vi "QueueDriver.vi"(0 "Queue Name":string, 5 "State":T2, 7 "State[]":T2[](array[typedef]), 11 "error in (no error)":errorcluster, 13 "Operations":T1) -> (4 "Dequeued Element":T2, 15 "error out":errorcluster)   [LabVIEW 2021]
doc: "This Vi acts a queue driver performing queue operations such as enqueue and dequeue."
uses:
  Controls/State.ctl
  Controls/Operations.ctl
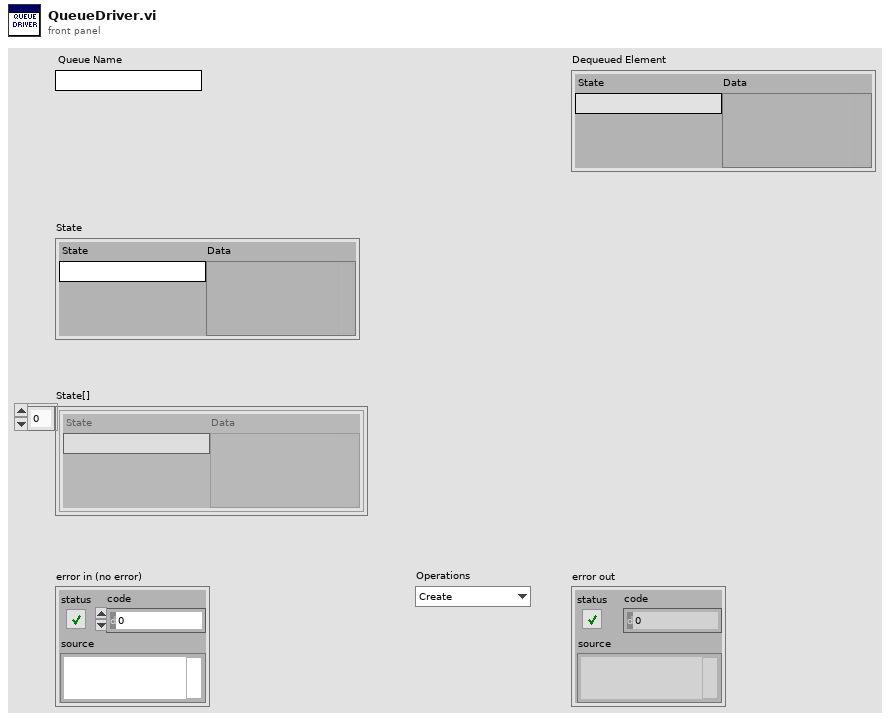
[diagram p1: front panel]
types:
  T1 = typedef "Operations.ctl" = enum16{"Create", "Enqueue", "Enqueue N", "Enstack", "Dequeue", "Flush", "Release"}
  T2 = typedef "State.ctl" = cluster{"State":string, "Data":variant}
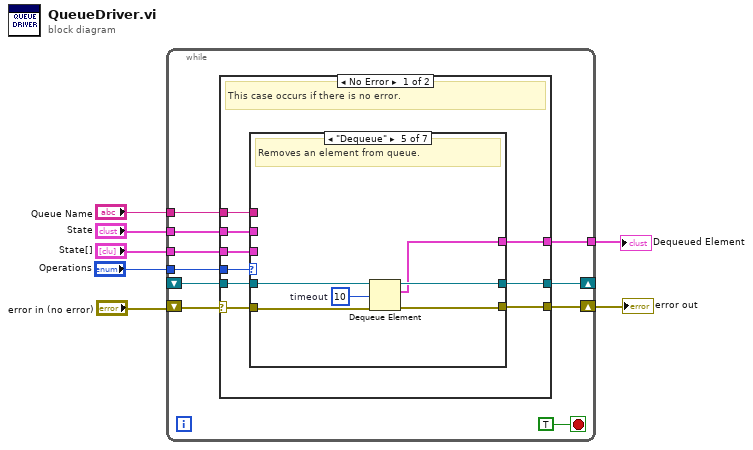
[diagram p0: block diagram]
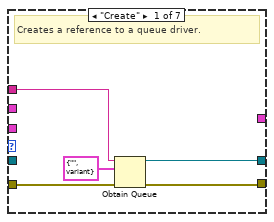
[diagram p2: hidden frame]
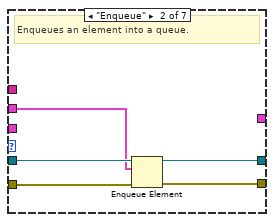
[diagram p3: hidden frame]
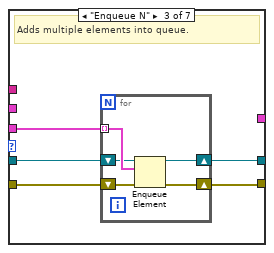
[diagram p4: hidden frame]
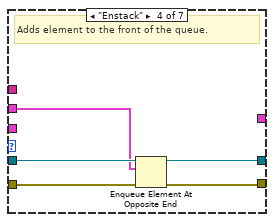
[diagram p5: hidden frame]
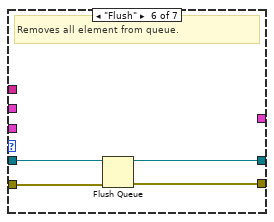
[diagram p6: hidden frame]
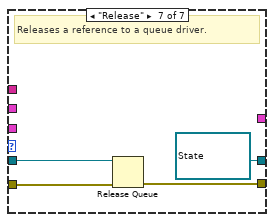
[diagram p7: hidden frame]
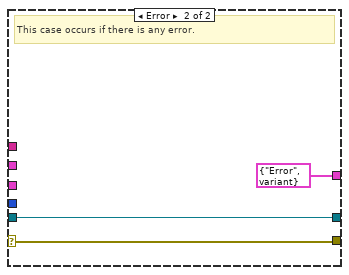
[diagram p8: hidden frame]
diagram:
  n1 = while {
    shift-right: [w12] -> w1
    shift-left: "error in (no error)" -> [w17]
    tunnel: "Operations" -> [w16]
    tunnel: "State[]" -> [w15]
    tunnel: "State" -> [w14]
    tunnel: "Queue Name" -> [w13]
    shift-right: [w11] -> _
    shift-left: _ -> [w10]
    tunnel: [w9] -> w2
    stop <- TRUE stop-if-true
    n2 = case shown="No Error" w17 {
      selector: w17 -> [w26 w68]
      tunnel: w16 -> [w25 _]
      tunnel: w15 -> [w24 _]
      tunnel: w14 -> [w23 _]
      tunnel: w13 -> [w22 _]
      tunnel: [w21 w68] -> w12
      tunnel: [w20 w66] -> w11
      tunnel: w10 -> [w19 w66]
      tunnel: [w18 T2 {"State"="Error", "Data"=variant} ("State")] -> w9
      frame No Error {
        # "This case occurs if there is no error."
        n3 = case shown="\"Dequeue\"" w25 {
          tunnel: w26 -> [w31 w36 w41 w51 w57 w61 w65]
          tunnel: w24 -> [_ _ w39 _ _ _ _]
          tunnel: w23 -> [_ w32 _ w48 _ _ _]
          tunnel: w22 -> [w29 _ _ _ _ _ _]
          tunnel: [w30 w35 w40 w50 w56 w60 w64] -> w21
          tunnel: [w27 w33 w37 w47 w53 w58 refnum<queue> refnum ("queue out")] -> w20
          tunnel: w19 -> [_ w34 w38 w49 w55 w59 w63]
          tunnel: [_ _ _ _ w52 _ _] -> w18
          frame "Create" {
            # "Creates a reference to a queue driver."
            n4 = Obtain Queue(name (unnamed)=w29, element data type=T2 {"State"="", "Data"=variant} ("State"), error in (no error)=w31) -> (queue out=w27:refnum<queue>, error out=w30:errorcluster)  [unwired: 2 in, 1 out]
          }
          frame "Enqueue" {
            # "Enqueues an element into a queue."
            n5 = Enqueue Element(queue=w34, element=w32, error in (no error)=w36) -> (queue out=w33:refnum<queue>, error out=w35:errorcluster)  [unwired: 1 in, 1 out]
          }
          frame "Enqueue N" {
            # "Adds multiple elements into queue."
            n6 = for {
              shift-right: [w45] -> w40
              shift-left: w41 -> [w46]
              tunnel: w39 -> [w44] mode=indexing
              shift-right: [w42] -> w37
              shift-left: w38 -> [w43]
              n7 = Enqueue Element(queue=w43, element=w44, error in (no error)=w46) -> (queue out=w42:refnum<queue>, error out=w45:errorcluster)  [unwired: 1 in, 1 out]
            }
          }
          frame "Enstack" {
            # "Adds element to the front of the queue."
            n8 = Enqueue Element At Opposite End(queue=w49, element=w48, error in (no error)=w51) -> (queue out=w47:refnum<queue>, error out=w50:errorcluster)  [unwired: 1 in, 1 out]
          }
          frame "Dequeue" {
            w54 = 10  # timeout
            # "Removes an element from queue."
            n9 = Dequeue Element(queue=w55, timeout in ms (-1)=w54, error in (no error)=w57) -> (queue out=w53:refnum<queue>, element=w52:T2, error out=w56:errorcluster)  [unwired: 1 out]
          }
          frame "Flush" {
            # "Removes all element from queue."
            n10 = Flush Queue(queue=w59, error in (no error)=w61) -> (queue out=w58:refnum<queue>, error out=w60:errorcluster)  [unwired: 1 out]
          }
          frame "Release" {
            # "Releases a reference to a queue driver."
            n11 = Release Queue(queue=w63, error in (no error)=w65) -> (error out=w64:errorcluster)  [unwired: 1 in, 2 out]
          }
        }
      }
      frame Error {
        # "This case occurs if there is any error."
      }
    }
  }
  "Dequeued Element" <- w2
  "error out" <- w1
